vi "StringifiedData.vi"(8 "error in (no error)":errorcluster, 11 "VariantMsg in":refnum<class "VariantMsg.lvclass">) -> (0 "error out":errorcluster, 2 "Stringified Data":string, 3 "VariantMsg out":refnum<class "VariantMsg.lvclass">)   [LabVIEW 2017, in "LapDog.Messaging.v3.NativeTypes.lvlib" / "VariantMsg.lvclass"]
doc: "This VI is used for the message probe. Child classes may override it and provide the message data in string format or a short string describing the data the message contains. This string will be displayed in the probe window."
uses:
  VariantMsg.lvclass
  VariantMsg.lvclass/VariantMsg.ctl
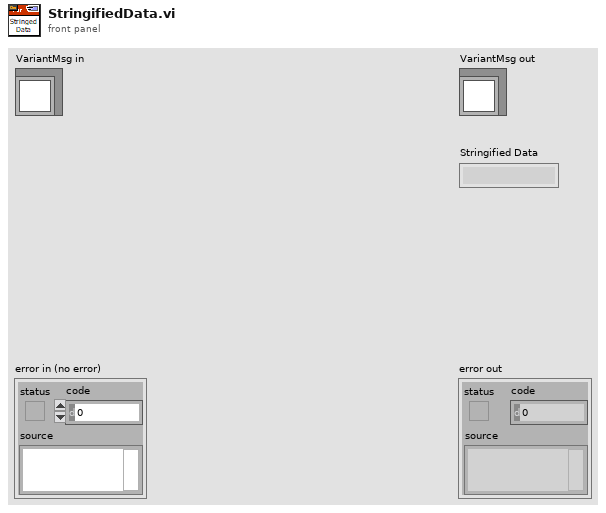
[diagram p1: front panel]
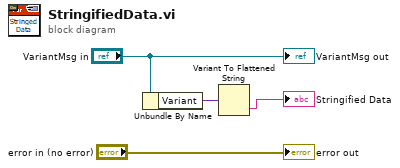
[diagram p0: block diagram]
diagram:
  n1 = Unbundle By Name("VariantMsg in") -> ("Variant"=w2:variant)
  n2 = Variant To Flattened String(Variant=w2) -> (data string=→"Stringified Data":string)  [unwired: 1 out]
  "error out" <- "error in (no error)"
  "VariantMsg out" <- "VariantMsg in"
